vi "DSF.Engine.Builder.Launch Thread.vi"(8 "error in (no error)":errorcluster, 10 "Thread Parameters":refnum<class "Thread Parameters.lvclass">, 11 "Builder in":refnum<class "DSF.Engine.Builder.lvclass">) -> (0 "error out":errorcluster, 3 "Builder out":refnum<class "DSF.Engine.Builder.lvclass">)   [LabVIEW 2017, in "DSF.Engine.lvlib" / "DSF.Engine.Builder.lvclass"]
uses:
  DSF.Engine.Builder.lvclass
  Thread Parameters/Thread Parameters.lvclass
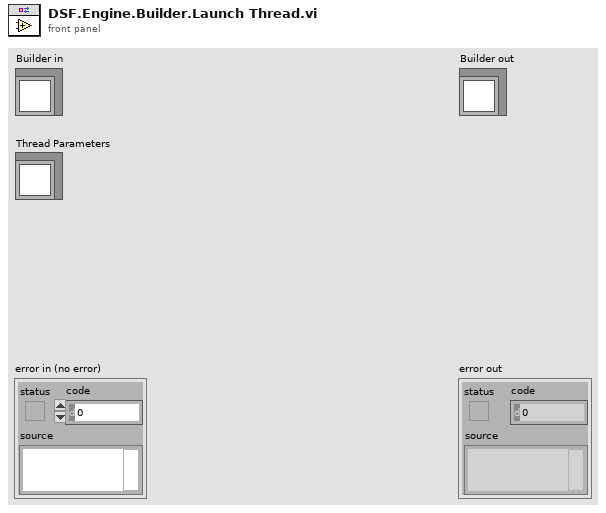
[diagram p1: front panel]
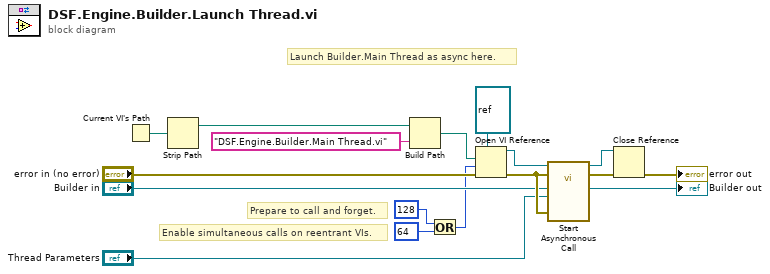
[diagram p0: block diagram]
diagram:
  # "Prepare to call and forget."
  # "Enable simultaneous calls on reentrant VIs."
  # "Launch Builder.Main Thread as async here."
  n1 = Current VI's Path() -> (path=w16:path)
  n2 = Strip Path(path=w16) -> (stripped path=w15:path)  [unwired: 1 out]
  n3 = Build Path(base path=w15, name or relative path="DSF.Engine.Builder.Main Thread.vi") -> (appended path=w8:path)
  n4 = Or(x=128 ("options"), y=64 ("options")) -> (x .or. y?=w2:i32)
  n5 = Open VI Reference(type specifier VI Refnum (for type only)=refnum<vi> refnum, vi path=w8, options=w2, error in (no error)="error in (no error)") -> (vi reference=w11:refnum<vi>, error out=w12:errorcluster)  [unwired: 2 in]
  n6 = call-by-ref "Start Asynchronous Call"(reference=w11, error in=w12, 8:"error in (no error)"=w12, "Thread Parameters"="Thread Parameters", "Builder in"="Builder in") -> (reference out=w9:refnum<vi>, error out=w10:errorcluster)  [unwired: 7 in, 2 out]
  n7 = Close Reference(reference=w9, error in (no error)=w10) -> (error out=→"error out":errorcluster)
  "Builder out" <- "Builder in"
